vi "LoadTest.vi"() -> ()   [LabVIEW 2012]
uses:
  <vilib>/Utility/file.llb/Write To Spreadsheet File (DBL).vi
panel:
  out "Array":dbl[](array[numeric])
  out "Waveform Chart":dbl(graph)
  out "error out":errorcluster
  in  "stop":bool
  in  "Gain":i32(ring)=1 items=["1"=1, "8"=2, "16"=3, "32"=4, "64"=5, "128"=6]
  in  "DataRate":i32(slide)=8 min=8 max=1000 step=8 scale=8.0..1000.0
  out "Converted Value":dbl
  out "Bridge Value (mV/V)":dbl
  in  "Channel":i32(ring) items=["0", "1", "2", "3"]
  out "# Bridges:":i32
  in  "Enable":bool
  out "Attached?":bool
  out "Serial Number":i32
  # "The increment should be 8 and coerced to the nearest digit."
  # "This example is designed for 1046"
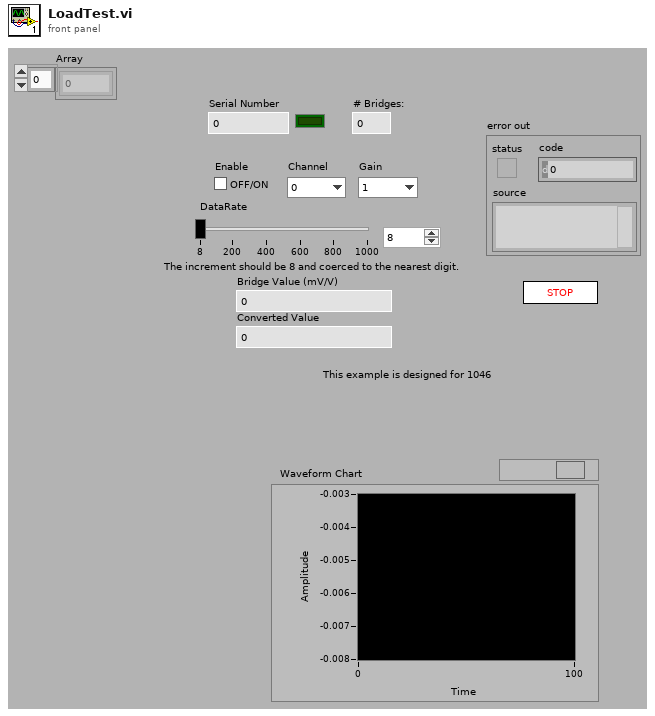
[diagram p1: front panel]
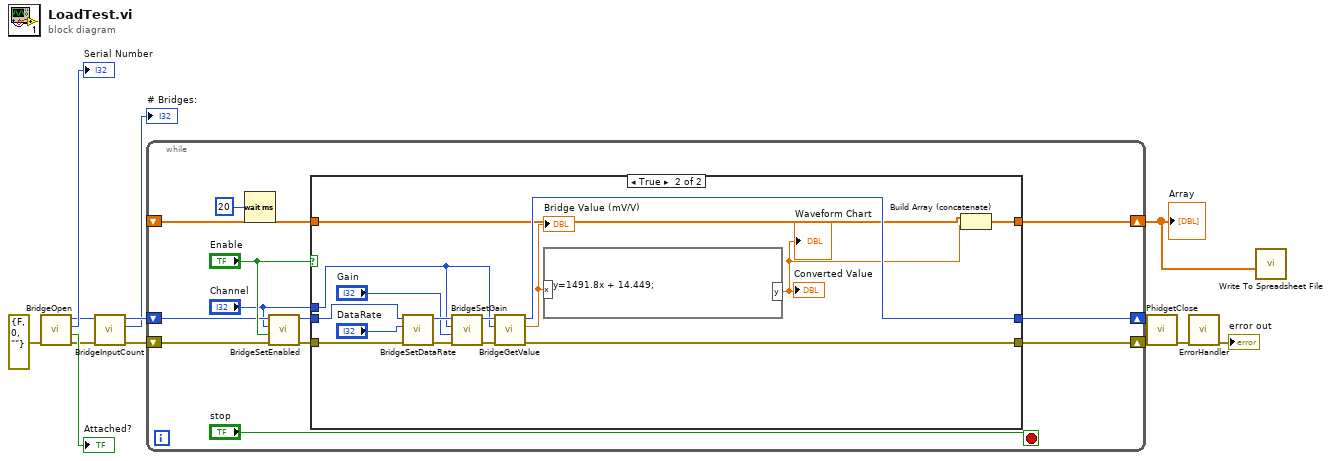
[diagram p0: block diagram]
diagram:
  n1 = call "BridgeOpen.vi"("error in (no error)"=errorcluster {"status"=FALSE, "code"=0, "source"=""}) -> ("error out"=w9:errorcluster, "Attached?"=→"Attached?":bool, "Serial Number Return"=→"Serial Number":i32, "Device Out"=w10:i32)  [unwired: 7 in]
  n2 = call "BridgeInputCount.vi"("error in (no error)"=w9, "Device In"=w10) -> ("error out"=w7:errorcluster, "Count"=→"# Bridges:":i32, "Device Out"=w8:i32)  [unwired: 7 in]
  n3 = while {
    shift-right: [w18] -> w5
    shift-left: w7 -> [w24]
    shift-right: [w19] -> w4
    shift-left: w8 -> [w22]
    shift-right: [w15] -> w1
    shift-left: _ -> [w14]
    stop <- "stop" stop-if-true
    n4 = Wait (ms)(milliseconds to wait=u32 20) -> ()  [unwired: 1 out]
    n5 = call "BridgeSetEnabled.vi"("error in (no error)"=w24, "SetEnabled"="Enable", "index"="Channel", "Device In"=w22) -> ("error out"=w23:errorcluster, "Device Out"=w21:i32)  [unwired: 5 in]
    n6 = case shown="True" "Enable" {
      tunnel: w21 -> [w28 w43]
      tunnel: w23 -> [w27 w37]
      tunnel: "Channel" -> [_ w40]
      tunnel: [w28 w36] -> w19
      tunnel: [w27 w35] -> w18
      tunnel: [w26 w30] -> w15
      tunnel: w14 -> [w26 w29]
      frame False {
      }
      frame True {
        # "calibration formula"
        n7 = call "BridgeSetDataRate.vi"("error in (no error)"=w37, "DataRate"="DataRate", "Device In"=w43) -> ("error out"=w38:errorcluster, "Device Out"=w42:i32)  [unwired: 6 in]
        n8 = call "BridgeSetGain.vi"("error in (no error)"=w38, "gain"="Gain", "index"=w40, "Device In"=w42) -> ("error out"=w39:errorcluster, "Device Out"=w41:i32)  [unwired: 5 in]
        n9 = call "BridgeGetValue.vi"("error in (no error)"=w39, "index"=w40, "Device In"=w41) -> ("error out"=w35:errorcluster, "value"=w34:dbl, "Device Out"=w36:i32)  [unwired: 5 in]
        "Bridge Value (mV/V)" <- w34
        n10 = formula code="y=1491.8x + 14.449;"("x"=w34) -> ("y"=w31:dbl)
        "Converted Value" <- w31
        "Waveform Chart" <- w31
        n11 = Build Array (concatenate)(w29, w31) -> (w30:dbl[])
      }
    }
  }
  "Array" <- w1
  n12 = call "PhidgetClose.vi"("error in"=w5, "Device In"=w4) -> ("error out"=w3:errorcluster)  [unwired: 9 in]
  n13 = call "ErrorHandler.vi"("error in"=w3) -> ("error out"=→"error out":errorcluster)  [unwired: 9 in, 1 out]
  n14 = call-poly <vilib>:"Write To Spreadsheet File.vi"("1D data"=w1) -> ()  [unwired: 7 in, 1 out]
